vi "VALEW_ATC_Verify Valve Time.vi"(7 "ATC Data":T1, 13 "T(target)":dbl) -> (6 "Pass/Fail?":bool, 8 "Report Text":string, 10 "Cold valve time (s) ATC":u16, 15 "Hot valve time (s) ATC":u16)   [LabVIEW 2016, in "2015 VA Washer.lvlib"]
uses:
  Projects/2015 VA Washer.lvlib
  typedefs/VALEW_ATC_Data.ctl
panel:
  out "Cold valve time (s) Calc":u16
  out "Hot valve time (s) Calc":u16
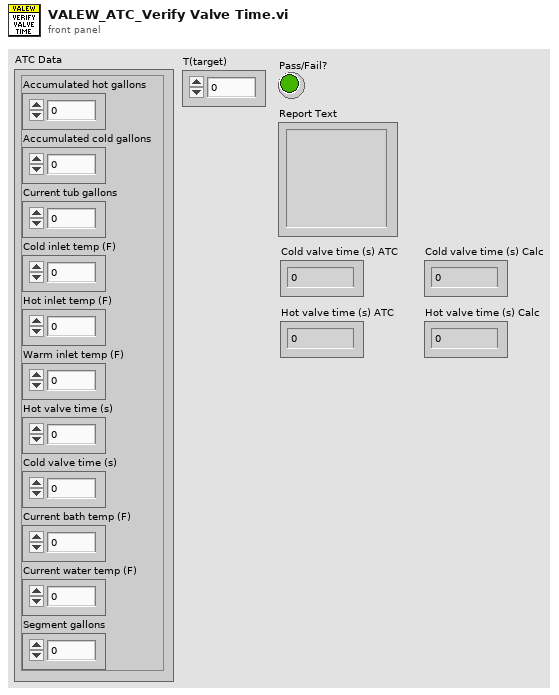
[diagram p1: front panel]
types:
  T1 = typedef "2015 VA Washer.lvlib/VALEW_ATC_Data.ctl" = cluster{"Accumulated hot gallons":dbl, "Accumulated cold gallons":dbl, "Current tub gallons":dbl, "Cold inlet temp (F)":dbl, "Hot inlet temp (F)":dbl, "Warm inlet temp (F)":dbl, "Hot valve time (s)":u16, "Cold valve time (s)":u16, "Current bath temp (F)":dbl, "Current water temp (F)":dbl, "Segment gallons":dbl}
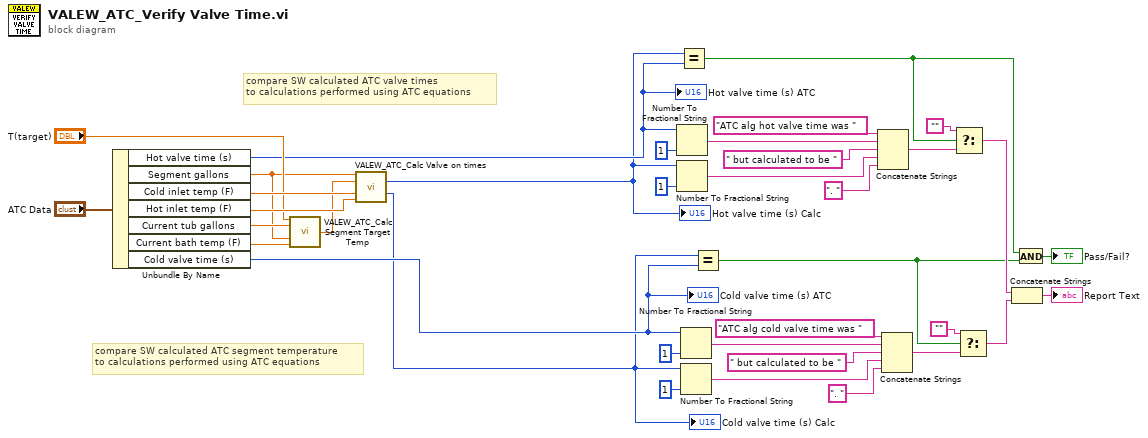
[diagram p0: block diagram]
diagram:
  # "compare SW calculated ATC valve times\nto calculations performed using ATC equations"
  # "compare SW calculated ATC segment temperature\nto calculations performed using ATC equations"
  n1 = Unbundle By Name("ATC Data") -> ("Hot valve time (s)"=w2:u16, "Segment gallons"=w6:dbl, "Cold inlet temp (F)"=w35:dbl, "Hot inlet temp (F)"=w36:dbl, "Current tub gallons"=w7:dbl, "Current bath temp (F)"=w5:dbl, "Cold valve time (s)"=w4:u16)
  "Cold valve time (s) ATC" <- w4
  "Hot valve time (s) ATC" <- w2
  n2 = call "VALEW_ATC_Calc Segment Target Temp.vi"("T(target)"="T(target)", "V(bath)"=w7, "V(segment)"=w6, "T(bath)"=w5) -> ("T(segment target)"=w34:dbl)  [unwired: 11 in]
  n3 = call "VALEW_ATC_Calc Valve on times.vi"("V(segment)"=w6, "T(segment target)"=w34, "T(cold inlet)"=w35, "T(hot inlet)"=w36) -> ("t(hot valve)"=w1:u16, "t(cold valve)"=w3:u16)  [unwired: 10 in]
  "Hot valve time (s) Calc" <- w1
  "Cold valve time (s) Calc" <- w3
  n4 = Number To Fractional String(number=w2, precision (6)=i16 1) -> (F-format string=w31:string)  [unwired: 2 in]
  n5 = Number To Fractional String(number=w1, precision (6)=i16 1) -> (F-format string=w29:string)  [unwired: 2 in]
  n6 = Equal?(x=w1, y=w2) -> (x = y?=w9:bool)
  n7 = Number To Fractional String(number=w4, precision (6)=i16 1) -> (F-format string=w20:string)  [unwired: 2 in]
  n8 = Number To Fractional String(number=w3, precision (6)=i16 1) -> (F-format string=w22:string)  [unwired: 2 in]
  n9 = Equal?(x=w3, y=w4) -> (x = y?=w8:bool)
  n10 = Concatenate Strings("ATC alg hot valve time was ", w31, " but calculated to be ", w29, ". " ("string")) -> (w26:string)
  n11 = Concatenate Strings("ATC alg cold valve time was ", w20, " but calculated to be ", w22, ". " ("string")) -> (w25:string)
  n12 = Select(t="", s=w9, f=w26) -> (s? t:f=w10:string)
  n13 = Select(t="", s=w8, f=w25) -> (s? t:f=w11:string)
  n14 = Concatenate Strings(w10, w11) -> (→"Report Text":string)
  n15 = And(x=w9, y=w8) -> (x .and. y?=→"Pass/Fail?":bool)
